vi "GlobalStop.vi"() -> ()   [LabVIEW 2018]
panel:
  in  "Гл.Стоп":bool
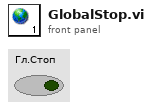
[diagram p1: front panel]
diagram:
